vi "testSubVI.vi"(8 "b":dbl, 11 "a":dbl) -> (2 "c":dbl)   [LabVIEW 2013]
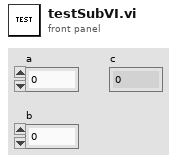
[diagram p1: front panel]
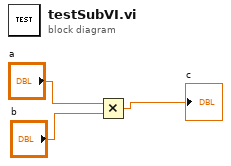
[diagram p0: block diagram]
diagram:
  n1 = Multiply(x="a", y="b") -> (x*y=→"c":dbl)
